vi "niSwitch Detach from Session.vi"(8 "error in":errorcluster, 10 "session in":variant, 11 "session factory in":refnum<class "Session Factory.lvclass">) -> (0 "error out":errorcluster)   [LabVIEW 2021, in "Session Management niSwitch.lvlib" / "Session Factory.lvclass"]
doc: "Detaches from the provided session."
uses:
  Session Factory.lvclass
  <vilib>/Plug-In SDKs/Sessions/Instrument/ISession Factory/Initialize and Close Session Behavior.ctl
  <vilib>/Plug-In SDKs/Sessions/Instrument/ISession Factory/ISession Factory.lvclass
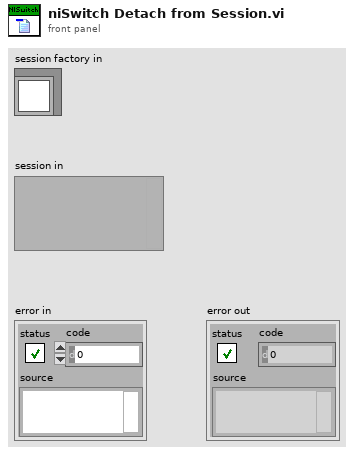
[diagram p1: front panel]
types:
  T1 = typedef "NI Session Management Instrument.lvlib/ISession Factory.lvclass/Initialize and Close Session Behavior.ctl" = enum16{"Initialize and Close", "Attach and Detach", "Initialize and Detach", "Attach and Close"}
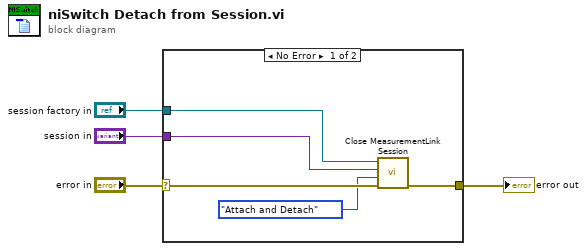
[diagram p0: block diagram]
diagram:
  n1 = case shown="No Error" "error in" {
    selector: "error in" -> [w9 w10]
    tunnel: [w8 w10] -> w4
    tunnel: "session in" -> [w7 _]
    tunnel: "session factory in" -> [w6 _]
    frame No Error {
      n2 = call-dynamic "Close MeasurementLink Session.vi"("error in"=w9, "initialize and close session behavior"=Initialize_and_Close_Session_Behavior."Attach and Detach", "session in"=w7, "session factory in"=w6) -> ("error out"=w8:errorcluster)  [unwired: 7 in]
    }
    frame Error {
    }
  }
  "error out" <- w4
